vi "ASI Set Control Value.vi"(7 "bAuto":i32, 9 "lValue":i32, 10 "ControlType":i32, 11 "iCameraID":i32) -> (3 "function return":i32)   [LabVIEW 2012, in "ASICamera2_no_err.lvlib"]
doc: "ASICAMERA_API ASI_ERROR_CODE ASISetControlValue(int iCameraID, ASI_CONTROL_TYPE ControlType, long lValue, ASI_BOOL bAuto);"
uses:
  <userlib>/ASICamera2_no_err/ASICamera2_no_err.lvlib
  ASICamera2.dll
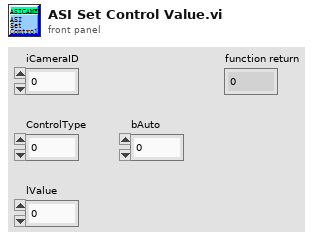
[diagram p1: front panel]
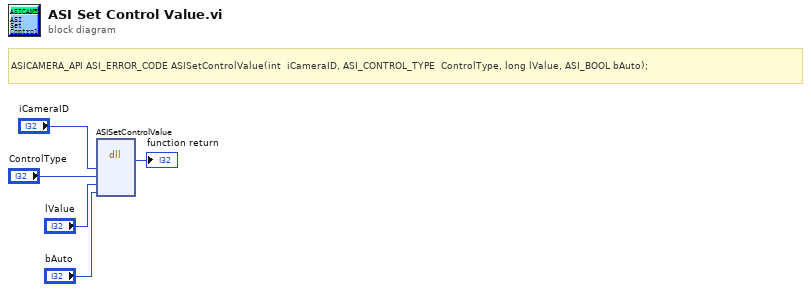
[diagram p0: block diagram]
diagram:
  # "ASICAMERA_API ASI_ERROR_CODE ASISetControlValue(int  iCameraID, ASI_CONTROL_TYPE  ControlType, long lValue, ASI_BOOL bAuto);"
  n1 = dll-call lib="ASICamera2.*" fn="ASISetControlValue"("iCameraID"="iCameraID", "ControlType"="ControlType", "lValue"="lValue", "bAuto"="bAuto") -> (→"function return":i32)  [unwired: 7 in, 2 out]
